vi "initFilename.vi"(1 "Experiment type":string(combo)="pumpprobe", 2 "Base disk and folder":string) -> (0 "folder name":string)   [LabVIEW 2017]
doc: "Initialize filename based on type of measurement and date and time."
uses:
  globalUtilities.vi
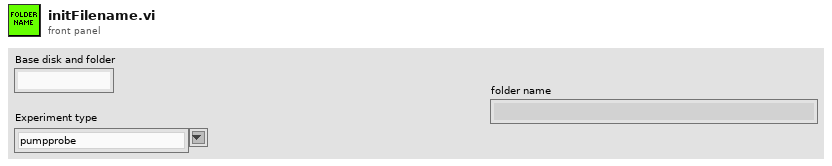
[diagram p1: front panel]
types:
  T1 = enum16{"open", "replace", "create", "open or create", "replace or create", "replace or create with confirmation"}
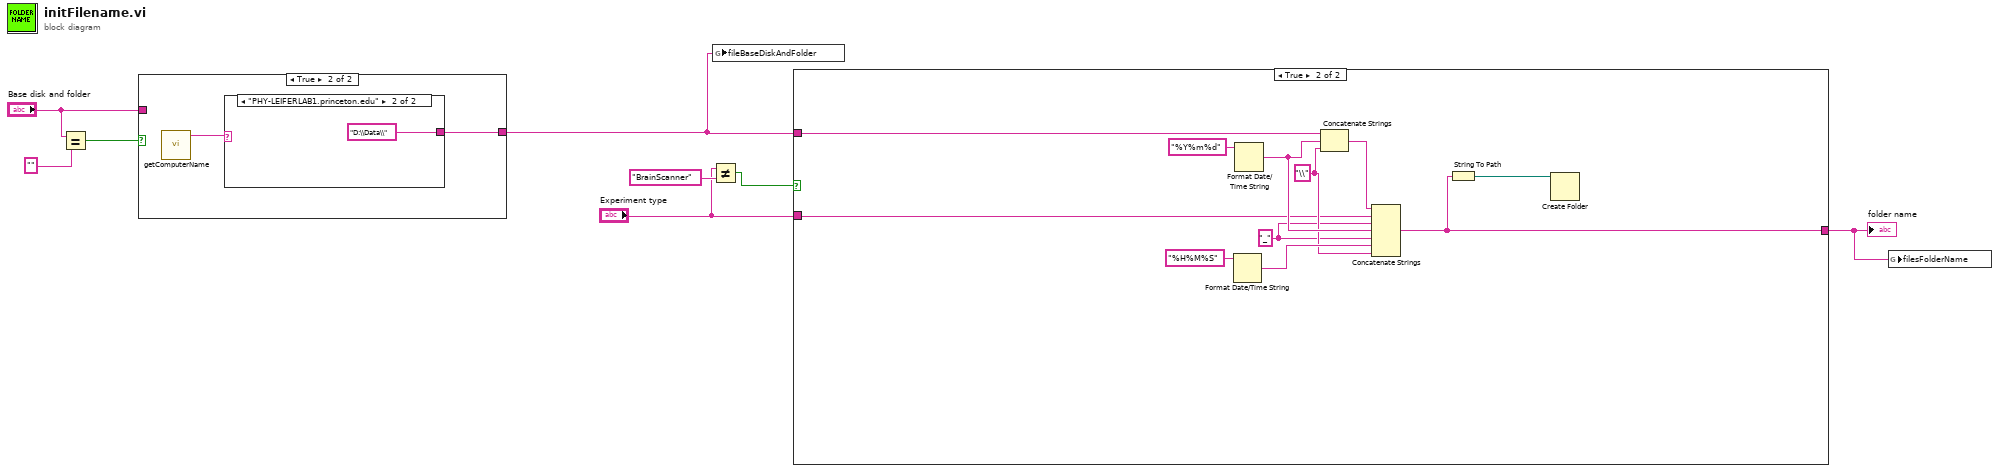
[diagram p0: block diagram]
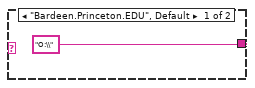
[diagram p3: hidden frame]
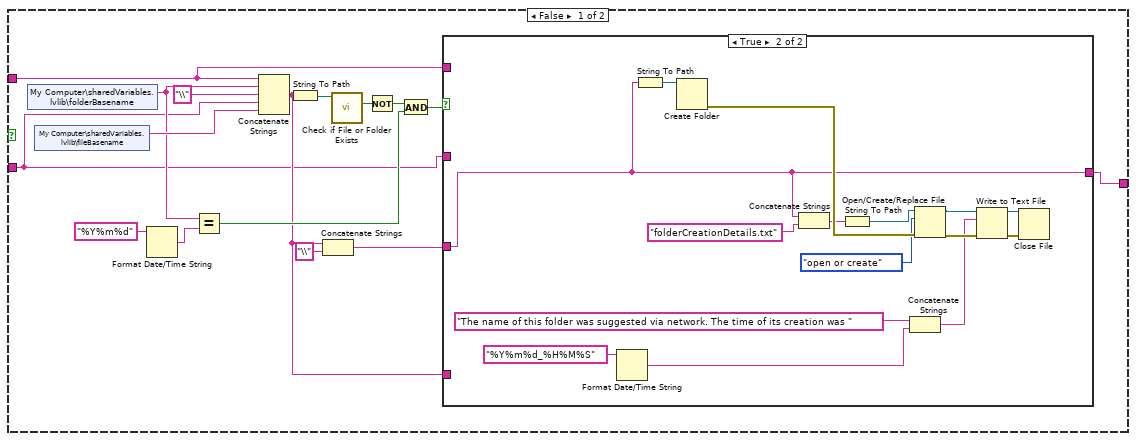
[diagram p4: hidden frame]
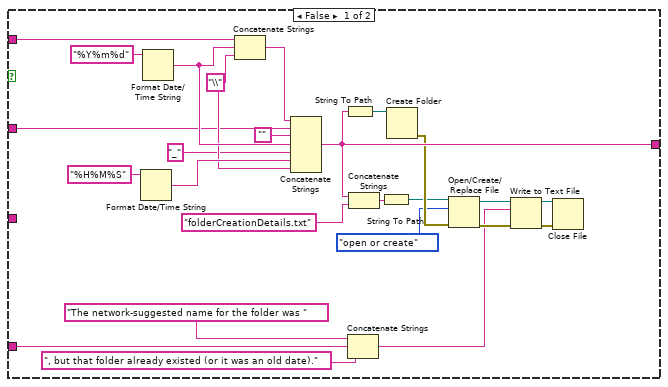
[diagram p5: hidden frame]
diagram:
  n1 = Equal?(x="Base disk and folder", y="") -> (x = y?=w3:bool)
  n2 = case shown="True" w3 {
    tunnel: [w9 w10] -> w2
    tunnel: "Base disk and folder" -> [w9 _]
    frame False {
    }
    frame True {
      n3 = call "getComputerName.vi"() -> ("full name"=w11:string)  [unwired: 1 in, 2 out]
      n4 = case shown="\"PHY-LEIFERLAB1.princeton.edu\"" w11 {
        tunnel: ["O:\\" "D:\\Data\\"] -> w10
        frame "Bardeen.Princeton.EDU", Default {
        }
        frame "PHY-LEIFERLAB1.princeton.edu" {
        }
      }
    }
  }
  n5 = Not Equal?(x="Experiment type", y="BrainScanner") -> (x != y?=w6:bool)
  n6 = global write "globalUtilities.vi" "fileBaseDiskAndFolder"(w2) -> ()
  n7 = case shown="True" w6 {
    tunnel: [w26 w74] -> w8
    tunnel: "Experiment type" -> [w14 w73]
    tunnel: w2 -> [w25 w72]
    frame False {
      n8 = shared-variable "My Computer\\sharedVariables.lvlib\\folderBasename"() -> (w16:string)  [unwired: 1 in, 1 out]
      n9 = shared-variable "My Computer\\sharedVariables.lvlib\\fileBasename"() -> (w28:string)  [unwired: 1 in, 1 out]
      n10 = Format Date/Time String(time format string (%c)="%Y%m%d") -> (date/time string=w23:string)  [unwired: 2 in]
      n11 = Equal?(x=w16, y=w23) -> (x = y?=w21:bool)
      n12 = Concatenate Strings(w25, w16, "\\" ("string"), w14, w28) -> (w15:string)
      n13 = String To Path(string=w15) -> (path=w27:path)
      n14 = Concatenate Strings(w15, "\\" ("string")) -> (w17:string)
      n15 = call <vilib>:"Check if File or Folder Exists.vi"("path"=w27) -> ("file or folder exists?"=w22:bool)  [unwired: 8 in, 2 out]
      n16 = Not(x=w22) -> (.not. x?=w19:bool)
      n17 = And(x=w19, y=w21) -> (x .and. y?=w20:bool)
      n18 = case shown="True" w20 {
        tunnel: [w44 w55] -> w26
        tunnel: w14 -> [w47 _]
        tunnel: w15 -> [w35 _]
        tunnel: w25 -> [w31 _]
        tunnel: w17 -> [_ w55]
        frame False {
          w49 = "\\"
          n19 = Format Date/Time String(time format string (%c)="%H%M%S") -> (date/time string=w53:string)  [unwired: 2 in]
          n20 = Format Date/Time String(time format string (%c)="%Y%m%d") -> (date/time string=w52:string)  [unwired: 2 in]
          n21 = Concatenate Strings(w31, w52, w49) -> (w54:string)
          n22 = Concatenate Strings(w54, w47, "", w52, "_", w53, w49) -> (w44:string)
          n23 = String To Path(string=w44) -> (path=w45:path)
          n24 = Concatenate Strings("The network-suggested name for the folder was " ("string"), w35, ", but that folder already existed (or it was an old date)." ("string")) -> (w32:string)
          n25 = Concatenate Strings(w44, "folderCreationDetails.txt") -> (w42:string)
          n26 = String To Path(string=w42) -> (path=w40:path)
          n27 = Create Folder(path (use dialog)=w45) -> (error out=w41:errorcluster)  [unwired: 2 in, 2 out]
          n28 = Open/Create/Replace File(file path (use dialog)=w40, error in=w41, operation (0:open)=T1."open or create") -> (refnum out=w39:refnum<file>, error out=w38:errorcluster)  [unwired: 3 in, 1 out]
          n29 = Write to Text File(file (use dialog)=w39, text=w32, error in=w38) -> (refnum out=w36:refnum<file>, error out=w37:errorcluster)  [unwired: 1 in, 1 out]
          n30 = Close File(refnum=w36, error in=w37) -> ()  [unwired: 2 out]
        }
        frame True {
          n31 = Format Date/Time String(time format string (%c)="%Y%m%d_%H%M%S") -> (date/time string=w58:string)  [unwired: 2 in]
          n32 = String To Path(string=w55) -> (path=w69:path)
          n33 = Create Folder(path (use dialog)=w69) -> (error out=w66:errorcluster)  [unwired: 2 in, 2 out]
          n34 = Concatenate Strings(w55, "folderCreationDetails.txt") -> (w64:string)
          n35 = String To Path(string=w64) -> (path=w63:path)
          n36 = Concatenate Strings("The name of this folder was suggested via network. The time of its creation was ", w58) -> (w57:string)
          n37 = Open/Create/Replace File(file path (use dialog)=w63, error in=w66, operation (0:open)=T1."open or create") -> (refnum out=w62:refnum<file>, error out=w67:errorcluster)  [unwired: 3 in, 1 out]
          n38 = Write to Text File(file (use dialog)=w62, text=w57, error in=w67) -> (refnum out=w61:refnum<file>, error out=w68:errorcluster)  [unwired: 1 in, 1 out]
          n39 = Close File(refnum=w61, error in=w68) -> ()  [unwired: 2 out]
        }
      }
    }
    frame True {
      w71 = "_"
      w76 = "\\"
      n40 = Format Date/Time String(time format string (%c)="%H%M%S") -> (date/time string=w77:string)  [unwired: 2 in]
      n41 = Format Date/Time String(time format string (%c)="%Y%m%d") -> (date/time string=w78:string)  [unwired: 2 in]
      n42 = Concatenate Strings(w72, w78, w76) -> (w75:string)
      n43 = Concatenate Strings(w75, w73, w71, w78, w71, w77, w76) -> (w74:string)
      n44 = String To Path(string=w74) -> (path=w70:path)
      n45 = Create Folder(path (use dialog)=w70) -> ()  [unwired: 2 in, 3 out]
    }
  }
  "folder name" <- w8
  n46 = global write "globalUtilities.vi" "filesFolderName"(w8) -> ()
